vi "Synthesize.vi"(0 "Moving Ripple Noise in":refnum<class "Moving Ripple Noise.lvclass">, 5 "Fs (Hz)":dbl, 7 "Npts":i32, 9 "Repetition":i32, 11 "error in (no error)":errorcluster) -> (4 "Moving Ripple Noise out":refnum<class "Moving Ripple Noise.lvclass">, 8 "Array":dbl[](array[numeric]), 15 "error out":errorcluster)   [LabVIEW 2020, in "Moving Ripple Noise.lvclass"]
uses:
  Moving Ripple Noise.lvclass
  Moving Ripple Noise.lvclass/Moving Ripple Noise.ctl
  Utility VIs/Math VIs/LinSpace (x0-dx-npts).vi
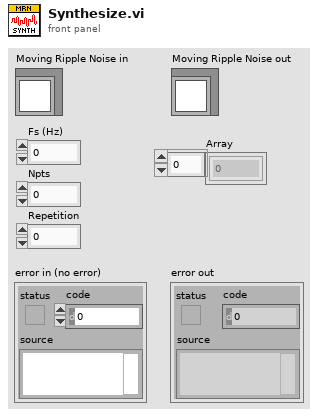
[diagram p1: front panel]
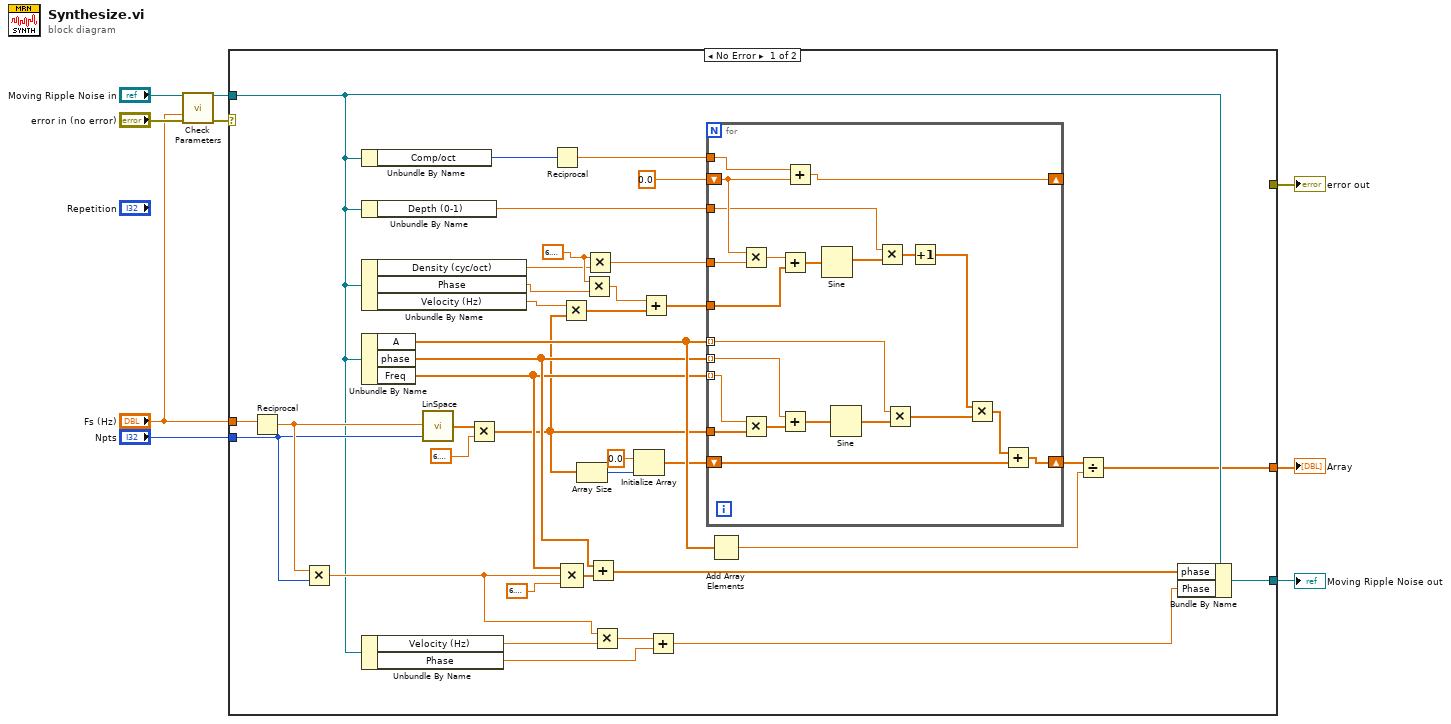
[diagram p0: block diagram]
diagram:
  n1 = call "Check Parameters.vi"("MRN in"="Moving Ripple Noise in", "Fs (Hz)"="Fs (Hz)", "error in (no error)"="error in (no error)") -> ("MRN out"=w4:refnum<class "Moving Ripple Noise.lvclass">, "error out"=w2:errorcluster)  [unwired: 11 in]
  n2 = case shown="No Error" w2 {
    selector: w2 -> [_ w69]
    tunnel: "Fs (Hz)" -> [w14 _]
    tunnel: "Npts" -> [w13 _]
    tunnel: w4 -> [w12 w70]
    tunnel: [w11 _] -> w8
    tunnel: [w10 w70] -> w7
    tunnel: [_ w69] -> w6
    frame No Error {
      w20 = 6.283185307179586
      n3 = Reciprocal(x=w14) -> (1/x=w34:dbl)
      n4 = Multiply(x=w34, y=w13) -> (x*y=w41:dbl)
      n5 = Unbundle By Name(w12) -> ("Comp/oct"=w28:i32)
      n6 = Unbundle By Name(w12) -> ("Depth (0-1)"=w30:dbl)
      n7 = Unbundle By Name(w12) -> ("Density (cyc/oct)"=w18:dbl, "Phase"=w19:dbl, "Velocity (Hz)"=w17:dbl)
      n8 = Unbundle By Name(w12) -> ("A"=w45:dbl[], "phase"=w39:dbl[], "Freq"=w35:dbl[])
      n9 = Unbundle By Name(w12) -> ("Velocity (Hz)"=w40:dbl, "Phase"=w43:dbl)
      n10 = call-poly "LinSpace.vi"("npts"=w13, "dx"=w34) -> ("Array"=w15:dbl[])  [unwired: 2 in, 1 out]
      n11 = Multiply(x=w15, y=6.283185307179586) -> (x*y=w31:dbl[])
      n12 = Reciprocal(x=w28) -> (1/x=w29:dbl)
      n13 = Multiply(x=w17, y=w31) -> (x*y=w25:dbl[])
      n14 = Compound Arithmetic op=MULTIPLY(w35, w41, 6.283185307179586) -> (w37:dbl[])
      n15 = Array Size(array=w31) -> (size(s)=w21:i32)
      n16 = Multiply(x=w20, y=w19) -> (x*y=w27:dbl)
      n17 = Multiply(x=w20, y=w18) -> (x*y=w23:dbl)
      n18 = Add(x=w39, y=w37) -> (x+y=w38:dbl[])
      n19 = Multiply(x=w41, y=w40) -> (x*y=w42:dbl)
      n20 = Initialize Array(0.0 ("element"), w21) -> (w32:dbl[])
      n21 = Add(x=w27, y=w25) -> (x+y=w26:dbl[])
      n22 = Add(x=w42, y=w43) -> (x+y=w44:dbl)
      n23 = for {
        tunnel: w45 -> [w52] mode=indexing
        tunnel: w23 -> [w68]
        shift-right: [w62] -> _
        shift-left: 0.0 -> [w64]
        tunnel: w26 -> [w66]
        tunnel: w29 -> [w63]
        tunnel: w30 -> [w60]
        tunnel: w31 -> [w58]
        tunnel: w39 -> [w55] mode=indexing
        tunnel: w35 -> [w57] mode=indexing
        shift-right: [w47] -> w33
        shift-left: w32 -> [w49]
        n24 = Multiply(x=w64, y=w68) -> (x*y=w67:dbl)
        n25 = Multiply(x=w57, y=w58) -> (x*y=w56:dbl[])
        n26 = Add(x=w67, y=w66) -> (x+y=w65:dbl[])
        n27 = Add(x=w55, y=w56) -> (x+y=w54:dbl[])
        n28 = Add(x=w63, y=w64) -> (x+y=w62:dbl)
        n29 = Sine(x=w65) -> (sin(x)=w61:dbl[])
        n30 = Sine(x=w54) -> (sin(x)=w53:dbl[])
        n31 = Multiply(x=w60, y=w61) -> (x*y=w59:dbl[])
        n32 = Multiply(x=w52, y=w53) -> (x*y=w51:dbl[])
        n33 = Increment(x=w59) -> (x+1=w50:dbl[])
        n34 = Multiply(x=w50, y=w51) -> (x*y=w48:dbl[])
        n35 = Add(x=w48, y=w49) -> (x+y=w47:dbl[])
      }
      n36 = Add Array Elements(numeric array=w45) -> (sum=w46:dbl)
      n37 = Divide(x=w33, y=w46) -> (x/y=w11:dbl[])
      n38 = Bundle By Name(cluster=w12, "phase"=w38, "Phase"=w44) -> (w10:refnum<class "Moving Ripple Noise.lvclass">)
    }
    frame Error {
    }
  }
  "error out" <- w6
  "Moving Ripple Noise out" <- w7
  "Array" <- w8
